vi "SPD Test Launcher.vi"() -> ()   [LabVIEW 2018]
uses:
  SPD Stand/typedefs/SPD.Stand Tabs.ctl
  SPD Stand/typedefs/SPD.Stand Ctrl.ctl
  Instruments/SPD HID Interface/hidSPDLibForLabView/LibVIs/hidSPD Controls/hidSPD Device Session.ctl
  Instruments/KC705 DevBoard/typedefs/DevB.Session.ctl
  Instruments/KeySight 53230A/typedefs/FreqC.Session.ctl
  Instruments/KeySight 8164B/KeySight 8164B LAN InstrLib/typedefs/KeySight 8164B control.ctl
  Instruments/SPD HID Interface/hidSPDLibForLabView/hidSPDLibForLabView.lvlib
  Instruments/KeySight 8164B/KeySight 8164B LAN InstrLib.lvlib
panel:
  out "test tabs":T1
  out "FreqC Selftest":bool caption="Пройдено"
  in  "FreqC Test":bool
  in  "HWCheck Conntction":bool
  out "spdDeviceSession.connected":bool caption="Детектор"
  out "DevBSession.connected":bool caption="КС705"
  out "8164BSession.connected":bool caption="8164B"
  out "FreqCSession.connected":bool caption="Частотомер"
  out "Console":string caption="Консоль"
  out "Error Out":errorcluster
  in  "stop":bool
  # "Расширенные тесты оборудования"
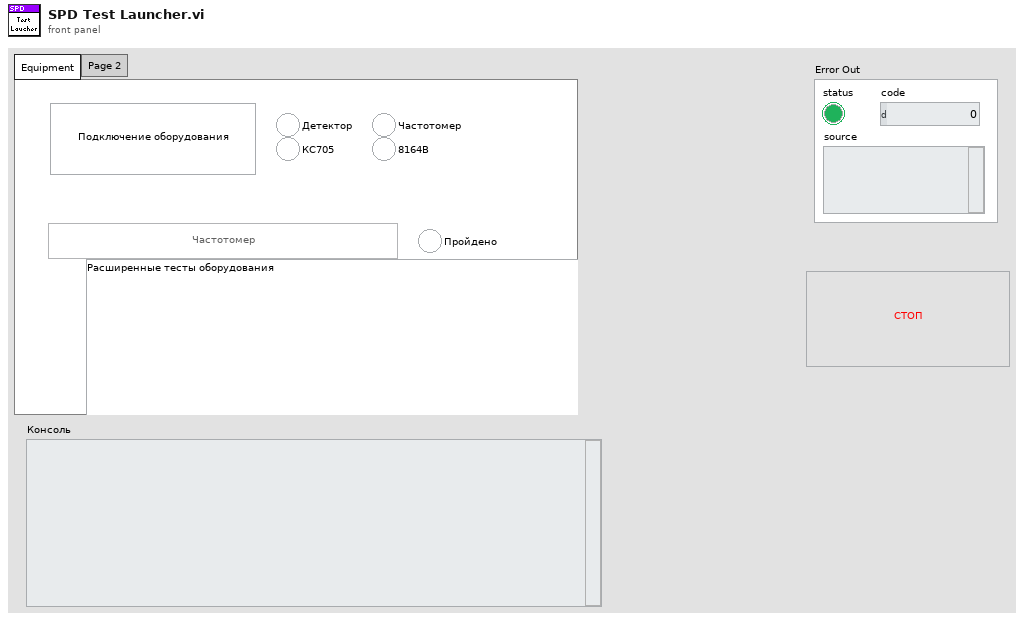
[diagram p1: front panel]
types:
  T1 = typedef "SPD.Stand Tabs.ctl" = enum32{"Equipment", "Page 2"}
  T2 = enum8{"Enabled", "Disabled", "Disabled and Grayed Out"}
  T3 = typedef "SPD.Stand Ctrl.ctl" = cluster{"spdDeviceSession":T4, "DevBSession":T5, "FreqCSession":T6, "8164BSession":T7}
  T4 = typedef "hidSPDLibForLabView.lvlib/hidSPD Device Session.ctl" = cluster{"spdRef":u64, "connected":bool}
  T5 = typedef "DevB.Session.ctl" = cluster{"DevBRef":refnum<visa-resource-name>, "connected":bool}
  T6 = typedef "FreqC.Session.ctl" = cluster{"FreqCRef":refnum<visa-resource-name>, "timeout":dbl, "connected":bool}
  T7 = typedef "KeySight 8164B LAN InstrLib.lvlib/KeySight 8164B control.ctl" = cluster{"Connection ID":refnum<k5>, "Connected":bool, "Info":string, "Slots Info":string[]}
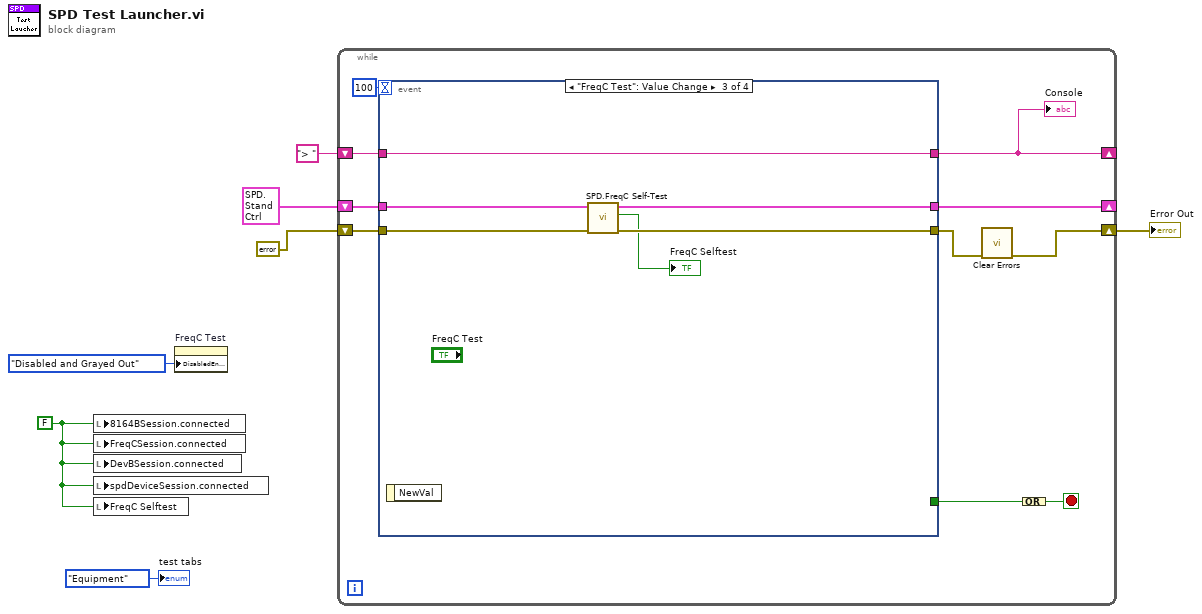
[diagram p0: block diagram]
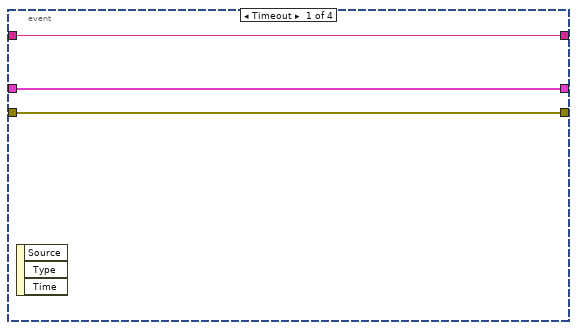
[diagram p2: hidden frame]
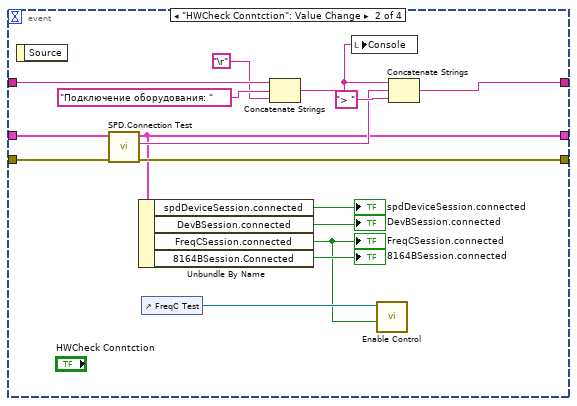
[diagram p3: hidden frame]
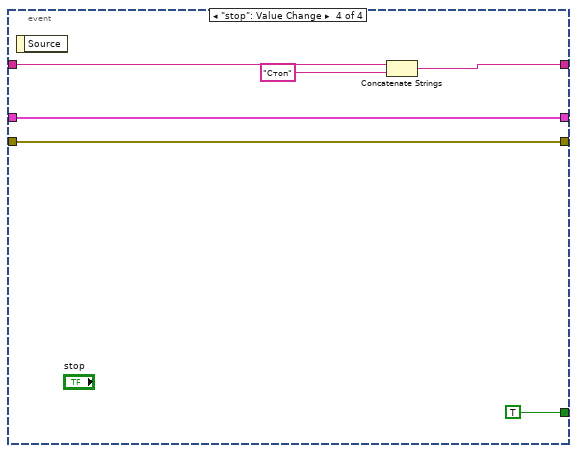
[diagram p4: hidden frame]
diagram:
  w2 = FALSE ("8164BSession.connected")
  n1 = local write "8164BSession.connected"(w2) -> ()
  n2 = local write "FreqCSession.connected"(w2) -> ()
  n3 = local write "DevBSession.connected"(w2) -> ()
  n4 = local write "spdDeviceSession.connected"(w2) -> ()
  n5 = local write "FreqC Selftest"(w2) -> ()
  n6 = property on="FreqC Test" class="Bool"("DisabledEnum"=T2."Disabled and Grayed Out" ("Disabled")) -> ()  [unwired: 2 in, 2 out]
  n7 = while {
    shift-right: [w15] -> _
    shift-left: T3 {"spdDeviceSession"={"spdRef"=0, "connected"=FALSE}, "DevBSession"={"DevBRef"="", "connected"=FALSE}, "FreqCSession"={"FreqCRef"="", "timeout"=0.0, "connected"=FALSE}, "8164BSession"={"Connection ID"=refnum, "Connected"=FALSE, "Info"="", "Slots Info"=[]}} ("SPD.Stand Ctrl") -> [w16]
    shift-right: [w8] -> w4
    shift-left: errorcluster {"status"=FALSE, "code"=0, "source"=""} ("Error In") -> [w14]
    shift-right: [w11] -> _
    shift-left: "> " ("string") -> [w12]
    stop <- w13 stop-if-true
    n8 = event shown="[2] \"FreqC Test\": Value Change" {
      selector: _ -> [_ _ _ _]
      dyn-events: _ -> [_ _ _ _]
      timeout: 100 -> [_ _ _ _]
      tunnel: [_ _ _ TRUE] -> w17
      tunnel: w16 -> [w20 w30 w41 w47]
      tunnel: [w20 w26 w38 w47] -> w15
      tunnel: w14 -> [w19 w29 w40 w46]
      tunnel: [w19 w28 w39 w46] -> w9
      tunnel: w12 -> [w18 w34 w42 w45]
      tunnel: [w18 w36 w42 w44] -> w11
      event Timeout {
        n9 = event-data() -> ()  [unwired: 1 in, 3 out]
      }
      event "HWCheck Conntction": Value Change {
        n10 = event-data() -> ()  [unwired: 1 in, 1 out]
        n11 = call "SPD.Connection Test.vi"("Error In"=w29, "SPD.Stand Ctrl in"=w30) -> ("Error Out"=w28:errorcluster, "HW report"=w27:string, "SPD.Stand Ctrl out"=w26:T3)  [unwired: 6 in, 1 out]
        n12 = Unbundle By Name(w26) -> ("spdDeviceSession.connected"=→"spdDeviceSession.connected":bool, "DevBSession.connected"=→"DevBSession.connected":bool, "FreqCSession.connected"=w21:bool, "8164BSession.Connected"=→"8164BSession.connected":bool)
        "FreqCSession.connected" <- w21
        n13 = control-ref of="FreqC Test"() -> (w22:refnum<vi>)
        n14 = Concatenate Strings(w34, "Подключение оборудования: " ("string"), "\r") -> (w32:string)
        n15 = local write "Console"(w32) -> ()
        n16 = call "Enable Control.vi"("enable"=w21, "Control"=w22) -> ()  [unwired: 10 in]
        n17 = Concatenate Strings(w32, w27, "> " ("string")) -> (w36:string)
      }
      event "FreqC Test": Value Change {
        n18 = event-data() -> ()  [unwired: 1 in, 1 out]
        n19 = call "SPD.FreqC Self-Test.vi"("Error In"=w40, "SPD.Stand Ctrl in"=w41) -> ("Error Out"=w39:errorcluster, "ok"=→"FreqC Selftest":bool, "SPD.Stand Ctrl out"=w38:T3)  [unwired: 7 in]
      }
      event "stop": Value Change {
        n20 = event-data() -> ()  [unwired: 1 in, 1 out]
        n21 = Concatenate Strings(w45, "Стоп" ("string")) -> (w44:string)
      }
    }
    "Console" <- w11
    n22 = call <vilib>:"Clear Errors.vi"("error in (no error)"=w9) -> ("error out"=w8:errorcluster)  [unwired: 5 in, 1 out]
    n23 = Compound Arithmetic op=OR(w17) -> (w13:bool)
  }
  "Error Out" <- w4
  "test tabs" <- SPD.Stand_Tabs."Equipment" ("test tabs")
